vi "Benchmark Read.vi"() -> ()   [LabVIEW 2017]
uses:
  Source/LookupTable/LookupTable.lvclass/LookupTable.ctl
  390d487d-10e4-4b9b-a12c-2aac0301551e.vi
  ed2deee6-b78a-453c-a366-a18b6818c8d7.vi
  Source/LookupTable/Read Table Reference.vi
  Source/LookupTable/LookupTable.lvclass
panel:
  in  "Table Size":i32=100000
  out "Array 3":i32[](array[numeric])
  out "Variant by reference":dbl
  out "Waveform Chart":cluster{dbl, dbl, dbl}(graph)
  out "Array 2":i32[](array[numeric])
  out "Array 1":i32[](array[numeric])
  out "Variant by value":dbl
  out "Composed Lookup Table":dbl
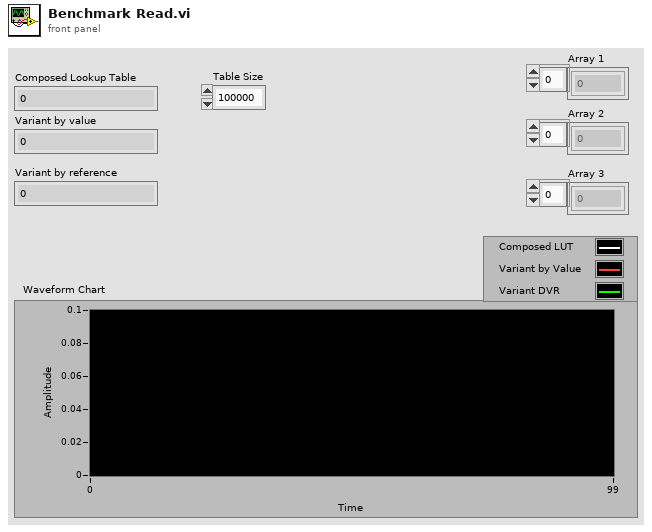
[diagram p1: front panel]
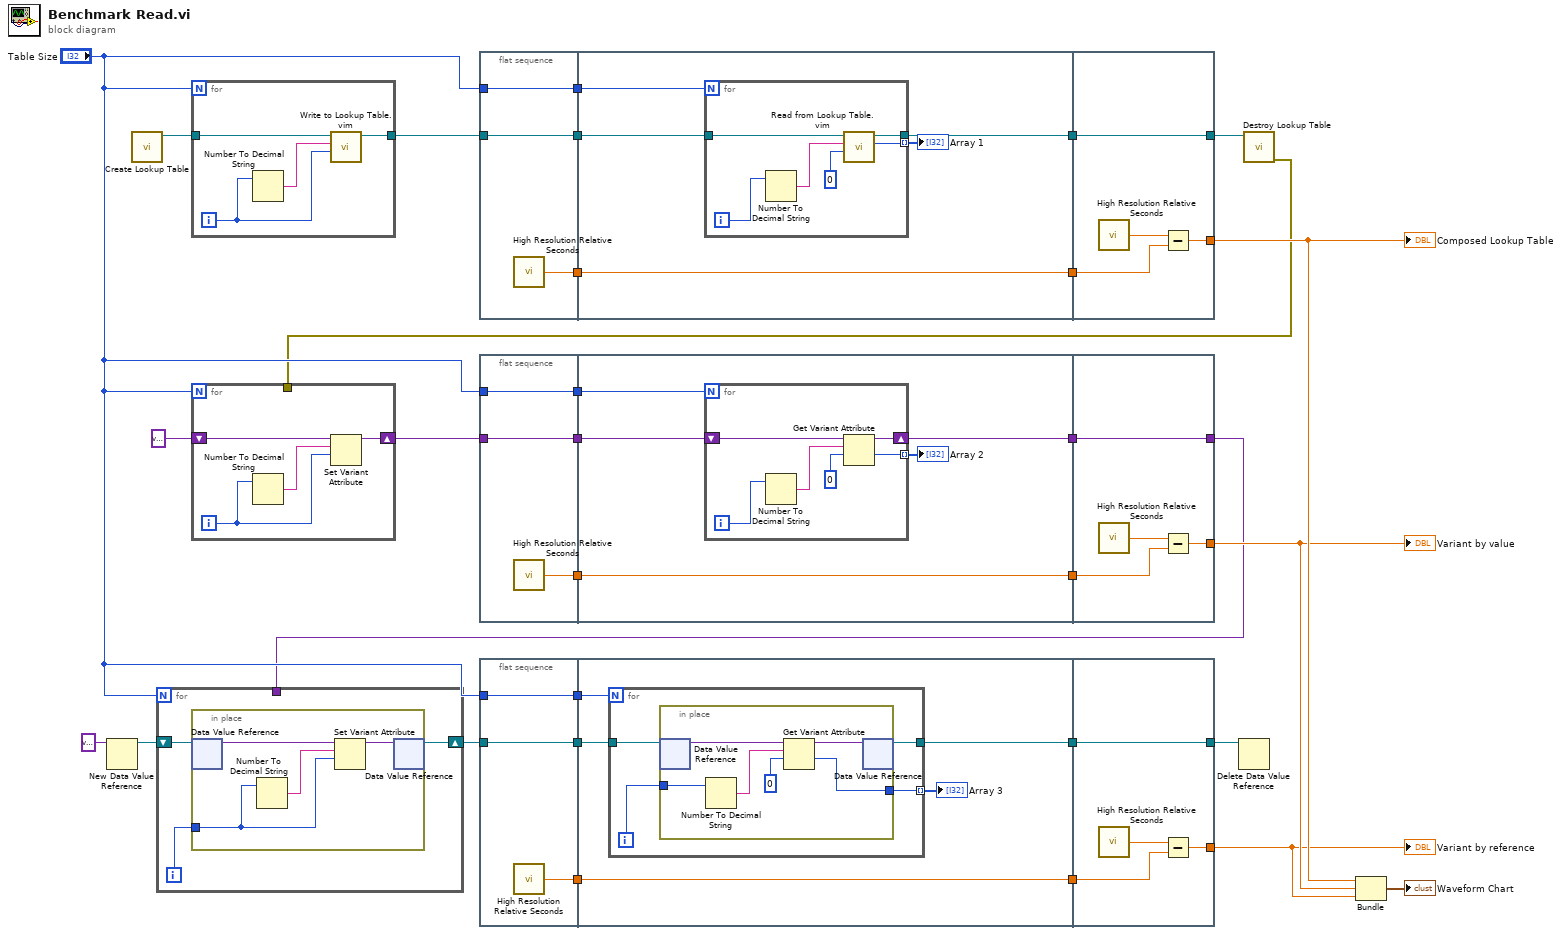
[diagram p0: block diagram]
diagram:
  n1 = New Data Value Reference(data value=variant) -> (data value reference=w10:refnum<data-value>)  [unwired: 1 in, 1 out]
  n2 = call "Create Lookup Table.vi"() -> ("LookupTable Reference"=w26:refnum<data-value>)  [unwired: 10 in, 1 out]
  n3 = for {
    N: "Table Size" -> [_]
    shift-right: [w33] -> w13
    shift-left: w10 -> [w34]
    tunnel: w2 -> [_]
    i -> [w32]
    n4 = in-place {
      in-place-border: w32 -> [w35]
      n5 = in-place-dvr #1(w34) -> (w37:variant)  [unwired: 1 out]
      n6 = Number To Decimal String(number=w35) -> (decimal integer string=w38:string)  [unwired: 1 in]
      n7 = Set Variant Attribute(Variant=w37, name=w38, value=w35) -> (Variant out=w36:variant)  [unwired: 1 in, 2 out]
      n8 = in-place-dvr #1(w36) -> (w33:refnum<data-value>)  [unwired: 1 out]
    }
  }
  n9 = for {
    N: "Table Size" -> [_]
    tunnel: [w40] -> w24
    tunnel: w26 -> [w39]
    i -> [w41]
    n10 = Number To Decimal String(number=w41) -> (decimal integer string=w42:string)  [unwired: 1 in]
    n11 = call "Write to Lookup Table.vim"("Item"=w41, "Item Name"=w42, "LookupTable Reference"=w39) -> ("LookupTable Reference Out"=w40:refnum<data-value>)  [unwired: 6 in, 2 out]
  }
  n12 = flat-sequence {
    tunnel: [w45] -> w31
    tunnel: [w44] -> w25
    tunnel: w24 -> [w44]
    tunnel: [w43] -> w19
    tunnel: "Table Size" -> [w43]
    tunnel: w31 -> [w50]
    tunnel: [w50] -> w30
    tunnel: w25 -> [w49]
    tunnel: [w48] -> w22
    tunnel: w19 -> [w47]
    tunnel: w30 -> [w59]
    tunnel: [w58] -> w7
    tunnel: [w57] -> w23
    tunnel: w22 -> [w57]
    frame #0 {
      n13 = call <vilib>:"High Resolution Relative Seconds.vi"() -> ("relative seconds"=w45:dbl)
    }
    frame #1 {
      n14 = for {
        N: w47 -> [_]
        tunnel: [w54] -> w48
        tunnel: w49 -> [w53]
        tunnel: [w51] -> w46 mode=indexing
        i -> [w55]
        n15 = Number To Decimal String(number=w55) -> (decimal integer string=w56:string)  [unwired: 1 in]
        n16 = call "Read from Lookup Table.vim"("Type"=0, "Item Name"=w56, "LookupTable Reference"=w53) -> ("Value"=w51:i32, "LookupTable Reference Out"=w54:refnum<data-value>)  [unwired: 5 in, 2 out]
      }
      "Array 1" <- w46
    }
    frame #2 {
      n17 = call <vilib>:"High Resolution Relative Seconds.vi"() -> ("relative seconds"=w60:dbl)
      n18 = Subtract(x=w60, y=w59) -> (x-y=w58:dbl)
    }
  }
  n19 = flat-sequence {
    tunnel: [w63] -> w29
    tunnel: [w62] -> w21
    tunnel: w20 -> [w62]
    tunnel: "Table Size" -> [w61]
    tunnel: [w61] -> w18
    tunnel: w29 -> [w68]
    tunnel: [w68] -> w28
    tunnel: w21 -> [w67]
    tunnel: w18 -> [w65]
    tunnel: [w64] -> w1
    tunnel: w28 -> [w77]
    tunnel: [w76] -> w6
    tunnel: [w75] -> w2
    tunnel: w1 -> [w75]
    frame #0 {
      n20 = call <vilib>:"High Resolution Relative Seconds.vi"() -> ("relative seconds"=w63:dbl)
    }
    frame #1 {
      n21 = for {
        N: w65 -> [_]
        shift-right: [w74] -> w64
        shift-left: w67 -> [w71]
        tunnel: [w69] -> w66 mode=indexing
        i -> [w72]
        n22 = Number To Decimal String(number=w72) -> (decimal integer string=w73:string)  [unwired: 1 in]
        n23 = Get Variant Attribute(Variant=w71, name=w73, default value (empty Variant)=0) -> (duplicate Variant=w74:variant, value=w69:i32)  [unwired: 1 in, 2 out]
      }
      "Array 2" <- w66
    }
    frame #2 {
      n24 = call <vilib>:"High Resolution Relative Seconds.vi"() -> ("relative seconds"=w78:dbl)
      n25 = Subtract(x=w78, y=w77) -> (x-y=w76:dbl)
    }
  }
  n26 = flat-sequence {
    tunnel: [w81] -> w17
    tunnel: [w80] -> w16
    tunnel: w13 -> [w80]
    tunnel: "Table Size" -> [w79]
    tunnel: [w79] -> w15
    tunnel: w17 -> [w86]
    tunnel: [w86] -> w14
    tunnel: w16 -> [w85]
    tunnel: w15 -> [w84]
    tunnel: [w82] -> w8
    tunnel: w14 -> [w99]
    tunnel: [w98] -> w5
    tunnel: [w97] -> w9
    tunnel: w8 -> [w97]
    frame #0 {
      n27 = call <vilib>:"High Resolution Relative Seconds.vi"() -> ("relative seconds"=w81:dbl)
    }
    frame #1 {
      n28 = for {
        N: w84 -> [_]
        tunnel: [w90] -> w83 mode=indexing
        tunnel: w85 -> [w88]
        tunnel: [w87] -> w82
        i -> [w89]
        n29 = in-place {
          in-place-border: [w94] -> w90
          in-place-border: w89 -> [w93]
          n30 = in-place-dvr #2(w88) -> (w92:variant)  [unwired: 1 out]
          n31 = Number To Decimal String(number=w93) -> (decimal integer string=w96:string)  [unwired: 1 in]
          n32 = Get Variant Attribute(Variant=w92, name=w96, default value (empty Variant)=0) -> (duplicate Variant=w91:variant, value=w94:i32)  [unwired: 1 in, 2 out]
          n33 = in-place-dvr #2(w91) -> (w87:refnum<data-value>)  [unwired: 1 out]
        }
      }
      "Array 3" <- w83
    }
    frame #2 {
      n34 = call <vilib>:"High Resolution Relative Seconds.vi"() -> ("relative seconds"=w100:dbl)
      n35 = Subtract(x=w100, y=w99) -> (x-y=w98:dbl)
    }
  }
  n36 = Delete Data Value Reference(data value reference=w9) -> ()  [unwired: 1 in, 2 out]
  n37 = call "Destroy Lookup Table.vi"("LookupTable Reference"=w23) -> ("error out"=w3:errorcluster)  [unwired: 10 in]
  n38 = for {
    N: "Table Size" -> [_]
    shift-right: [w104] -> w20
    shift-left: variant -> [w101]
    tunnel: w3 -> [_]
    i -> [w102]
    n39 = Number To Decimal String(number=w102) -> (decimal integer string=w103:string)  [unwired: 1 in]
    n40 = Set Variant Attribute(Variant=w101, name=w103, value=w102) -> (Variant out=w104:variant)  [unwired: 1 in, 2 out]
  }
  n41 = Bundle(w7, w6, w5) -> (→"Waveform Chart":cluster{dbl, dbl, dbl})  [unwired: 1 in]
  "Composed Lookup Table" <- w7
  "Variant by value" <- w6
  "Variant by reference" <- w5
